vi "AlazarGetBoardBySystemId.vi"(3 "error in (no error)":errorcluster, 4 "Board ID":u32=1, 5 "System ID":u32=1) -> (0 "error out":errorcluster, 1 "Return Code":u32, 2 "Handle":u32)   [LabVIEW 2021]
doc: "Get a handle to a board in a board system where the board system is specified its system identifier and the board by its board identifier within the board system."
uses:
  ATSApi.dll
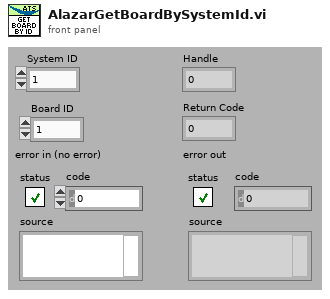
[diagram p1: front panel]
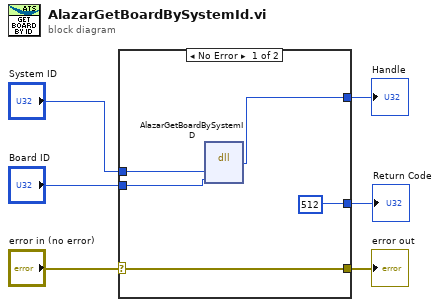
[diagram p0: block diagram]
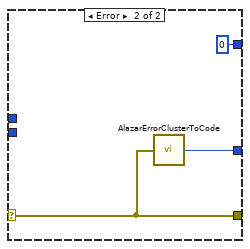
[diagram p2: hidden frame]
diagram:
  n1 = case shown="No Error" "error in (no error)" {
    selector: "error in (no error)" -> [w8 w14]
    tunnel: [w8 w14] -> w5
    tunnel: "System ID" -> [w11 _]
    tunnel: [w9 u32 0] -> w3
    tunnel: "Board ID" -> [w10 _]
    tunnel: [512 w13] -> w1
    frame No Error {
      n2 = dll-call lib="ATSApi.dll" fn="AlazarGetBoardBySystemID"("systemID"=w11, "boardID"=w10) -> (w9:u32)  [unwired: 5 in, 2 out]
    }
    frame Error {
      n3 = call "AlazarErrorClusterToCode.vi"("error in (no error)"=w14) -> ("Error Code"=w13:u32)
    }
  }
  "Handle" <- w3
  "error out" <- w5
  "Return Code" <- w1
